vi "LWXPS_INTServitudesStatusGet.vi"(0 "XPS Reference IN":refnum<k24>, 11 "LabVIEW error IN":errorcluster) -> (4 "XPS Reference OUT":refnum<k24>, 6 "Returned error code":i32, 8 "INT Servitudes Status":i16, 10 "XPS Error String":string, 15 "LabVIEW error OUT":errorcluster)   [LabVIEW 2014]
uses:
  D:/XPSQ8_LabView_Library/Development/Source/Dll/Newport.XPS.CommandInterface.dll
  Dll/Newport.XPS.CommandInterface.dll
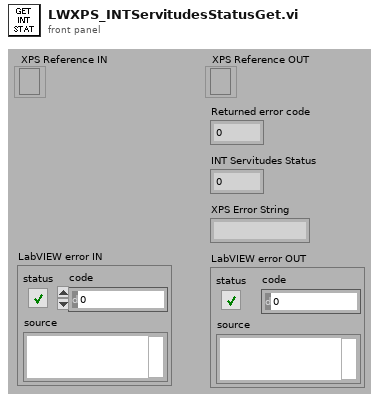
[diagram p1: front panel]
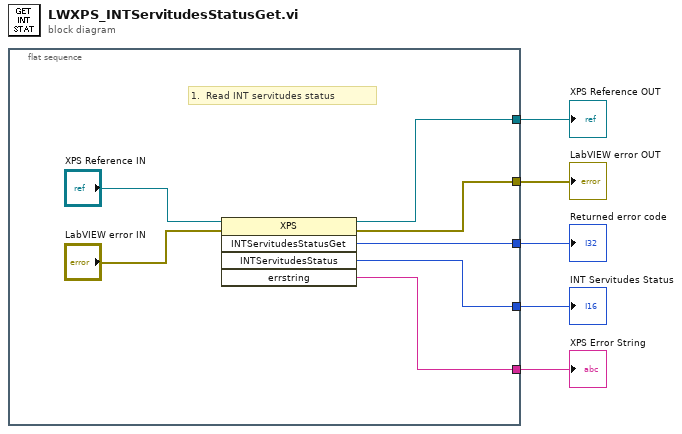
[diagram p0: block diagram]
diagram:
  n1 = flat-sequence {
    tunnel: [w10] -> w5
    tunnel: [w12] -> w4
    tunnel: [w9] -> w3
    tunnel: [w8] -> w1
    tunnel: [w6] -> w2
    frame #0 {
      # "1.  Read INT servitudes status"
      n2 = invoke class="XPS" method="INTServitudesStatusGet"(reference="XPS Reference IN", error in="LabVIEW error IN") -> (reference out=w10:refnum<k24>, error out=w12:errorcluster, "INTServitudesStatusGet"=w9:i32, "INTServitudesStatus"=w8:i16, "errstring"=w6:string)  [unwired: 3 in]
    }
  }
  "XPS Reference OUT" <- w5
  "LabVIEW error OUT" <- w4
  "Returned error code" <- w3
  "XPS Error String" <- w2
  "INT Servitudes Status" <- w1
